vi "xy_stack_setup.vi"() -> ()   [LabVIEW 2016]
uses:
  xy_stack_global.vi
  MotorPosition.vi
panel:
  out "index 4":i32
  out "index 3":i32
  out "index 2":i32
  out "index 1":i32
  out "Array 2":bool[](array[boolean])
  in  "compareFOV":bool
  out "xLoc ROI":dbl
  out "yLoc ROI":dbl
  in  "LoadROIinfo":bool
  out "Image 2":dbl[][](graph)
  out "size(s)":i32[](array[numeric])
  in  "SaveROI":bool
  out "loading data":bool
  in  "LoadFOV":bool
  in  "String 4":string
  in  "String 3":string
  in  "String 2":string
  in  "String":string
  in  "String":string
  in  "go 5":bool
  out "save 1 y 5":dbl
  out "save 1 x 5":dbl
  in  "save 5":bool
  in  "go 4":bool
  out "save 1 y 4":dbl
  out "save 1 x 4":dbl
  in  "save 4":bool
  in  "go 3":bool
  out "save 1 y 3":dbl
  out "save 1 x 3":dbl
  in  "save 3":bool
  in  "go 2":bool
  out "save 1 y 2":dbl
  out "save 1 x 2":dbl
  in  "save 2":bool
  in  "go 1":bool
  out "save 1 y":dbl
  out "save 1 x":dbl
  in  "save 1":bool
  in  "Current MIN":bool
  out "Scan Origin":cluster{dbl, dbl}
  in  "Step Size from BS FOV":bool
  in  "Image Flipped":bool
  in  "Step Xmin":bool
  in  "Step Ymax":bool
  in  "Step Ymin":bool
  in  "Step Xmax":bool
  in  "Current MAX":bool
  in  "save":bool
  in  "update":bool
  in  "Stage to cursor":bool
  in  "New XY limits":bool
  in  "BeamScanner Scanning":bool
  out "Size new Frame":i32[](array[numeric])
  out "size array init":i32[](array[numeric])
  out "size Array IN":i32[](array[numeric])
  out "size array out":i32[](array[numeric])
  out "Frame No":u16
  in  "Latest Frame":dbl[][](array[numeric])
  out "FOV Frame":dbl(ring)=64.0 items=["4x4 µm"=0.01860032550569635, "8x8 µm"=0.0372006510113927, "16x16 µm"=0.0744013020227854, "32x32 µm"=0.1488026040455708, "64x64 µm"=0.2976052080911416, "128x128 µm"=0.5952104161822832, "256x256 µm"=1.1904208323645664, "512x512 µm"=2.380841664729133, "1024x1024 µm"=4.761683329458266, "0x0"=0.0]
  out "No. Pixels Frame":i32(ring)=128 items=["8x8"=8, "16x16"=16, "32x32"=32, "64x64"=64, "128x128"=128, "256x256"=256, "512x512"=512, "1024x1024"=1024, "optimal"=1014]
  in  "Warning Limits":dbl[][](array[numeric])=[[5000.0], [5000.0]]
  in  "Safety Limits":dbl[][](array[numeric])=[[10000.0, 100000.0], [12000.0, 62000.0]]
  in  "Write Protection":bool
  out "Image":dbl[][](graph)
  out "Travel time short":dbl
  out "Travel time long":dbl
  in  "Acceleration":dbl=10000.0 format="%#_8g"
  in  "MAX Speed":dbl=1000.0
  in  "exit":bool
  out "requested y-position":dbl=35000.0
  out "requested x-position":dbl=35000.0
  in  "Move to Y":bool
  in  "Move to X":bool
  out "# steps Y":u16=20 step=1 format="%#.0f"
  in  "Y-Maximum":dbl=35000.0 min=12000.0 max=62000.0 format="%#.2f"
  in  "Y-Minimum":dbl=33849.9 min=12000.0 max=62000.0 format="%#.2f"
  in  "Step size Y":dbl=60.0 min=0.0
  out "Y-Position":sgl format="%.2f"
  out "# steps X":u16=20 step=1 format="%#.0f"
  in  "X-Maximum":dbl=38037.9 min=10000.0 max=100000.0 format="%#.2f"
  in  "X-Minimum":dbl=38037.9 min=10000.0 max=100000.0 format="%#.2f"
  in  "Step size X":dbl=60.0 min=0.0
  out "X-Position":sgl format="%.2f"
  # "9000px * 9000 px = 4GB Ram ca, test if clever saving needed"
  # "Check velocities in KINESIS: MAYBE 10000µm/s and 100000µm/s^2"
  # "Beamscanner Settings"
  # "dX relative to start"
  # "Xmin, Xmax"
  # "SETUP"
  # "Ymin, Ymax"
  # "dY relative to start"
  # "!!! Arbitrary, assumes Objective is centrally)\n(Objective Might leave Microscope Slide/Petri Dish)"
  # "Enter values from Kinesis \nto calculate imaging delay"
  # "(Objective would touch frame)"
  # "(automatic)"
  # "µm/s^2"
  # "µm/s"
  # "x"
  # "Cursors"
  # "y"
  # "Variables"
  # "Debugging"
  # "training data: \ncalc non-spectrally-imaged frames"
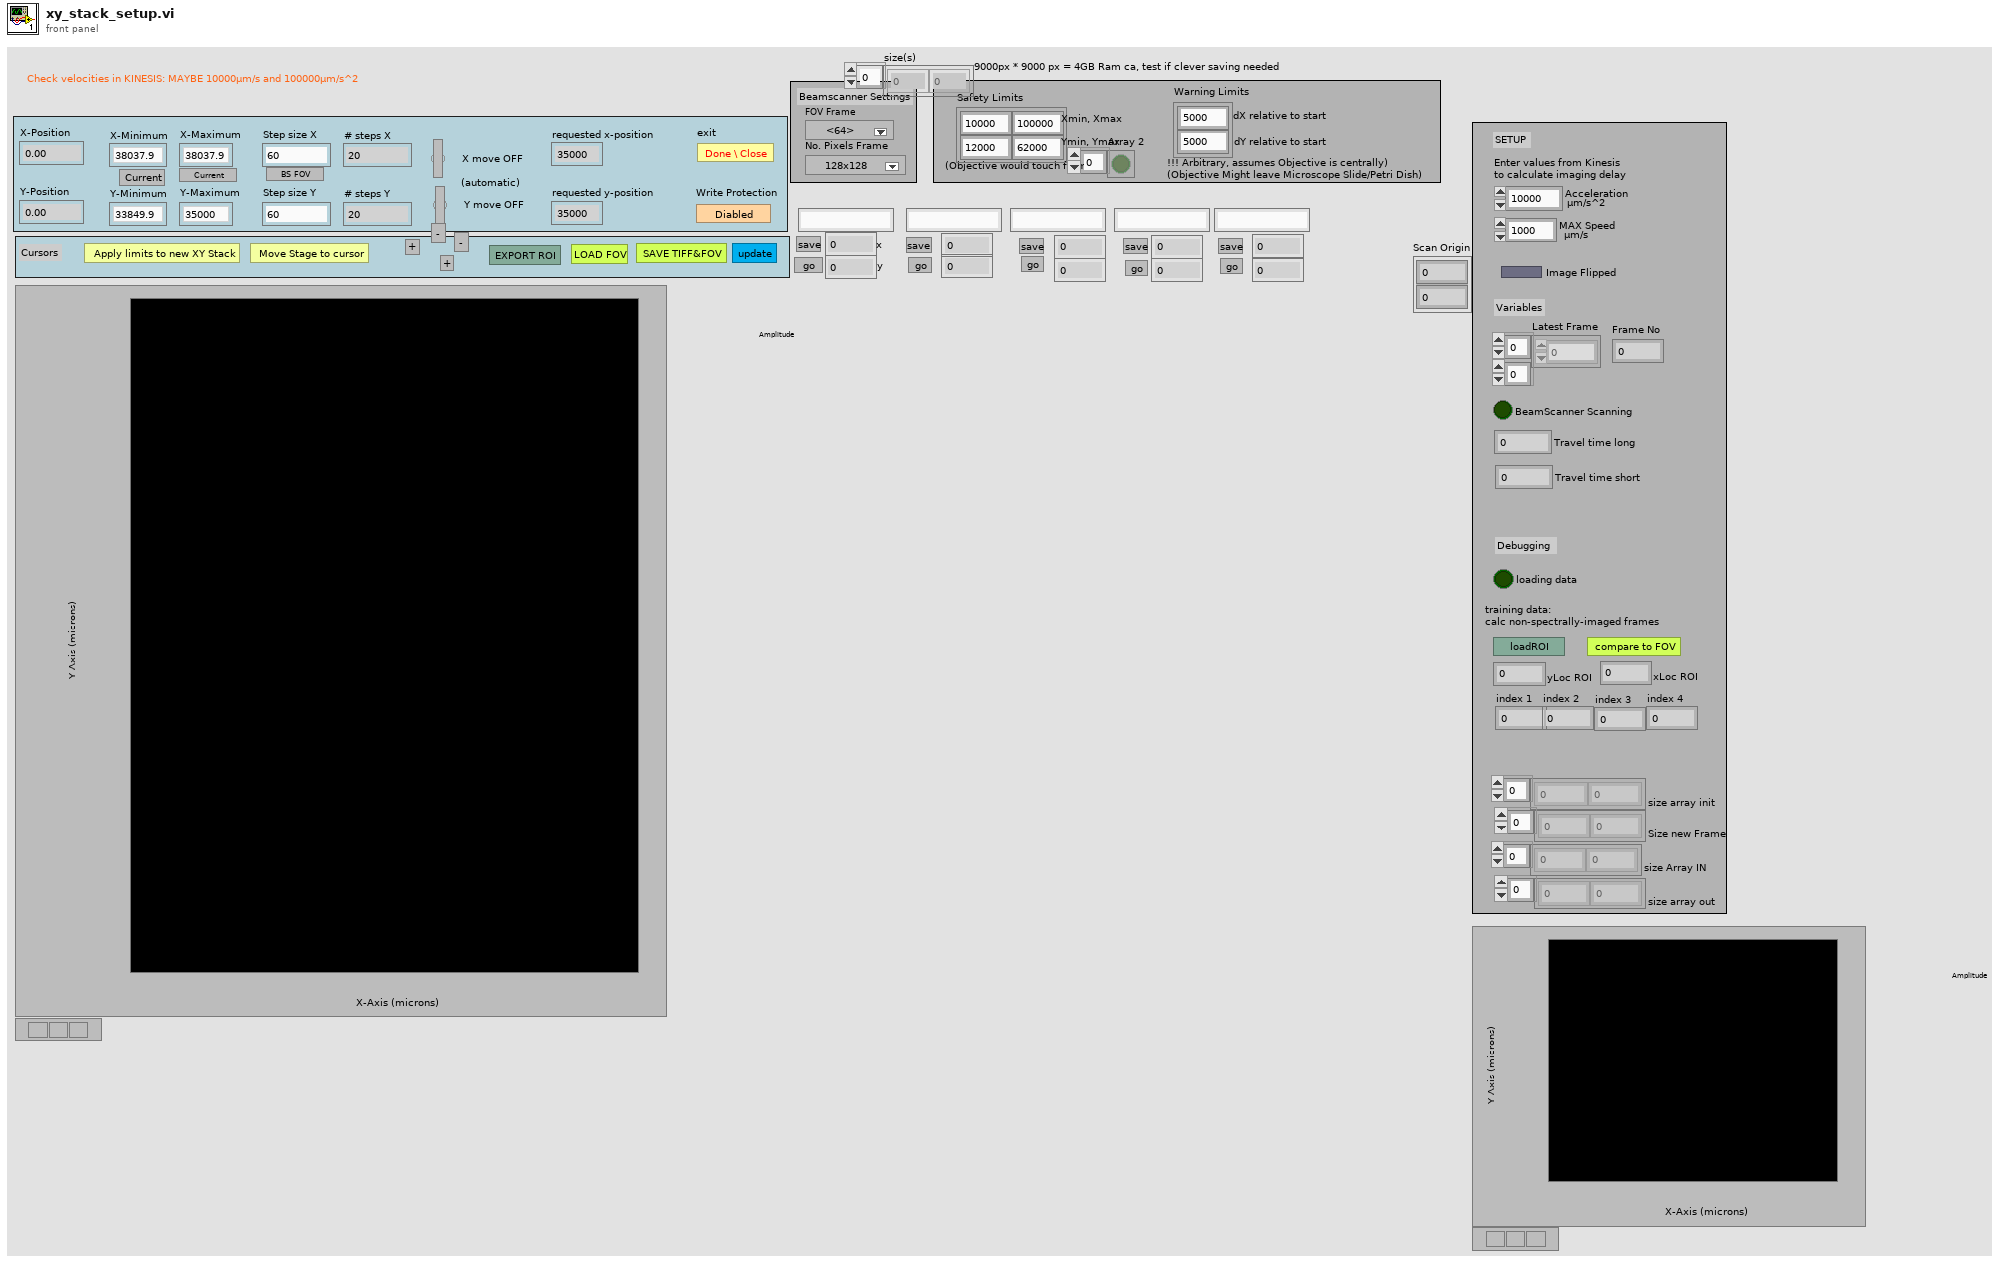
[diagram p1: front panel]
types:
  T1 = cluster{"Rows Per Strip":i32, "Photometric":i32, "Compression Type":i32}
  T2 = typedef "Image Type" = u32
  T3 = typedef "IMAQ Image.ctl" = refnum<image>
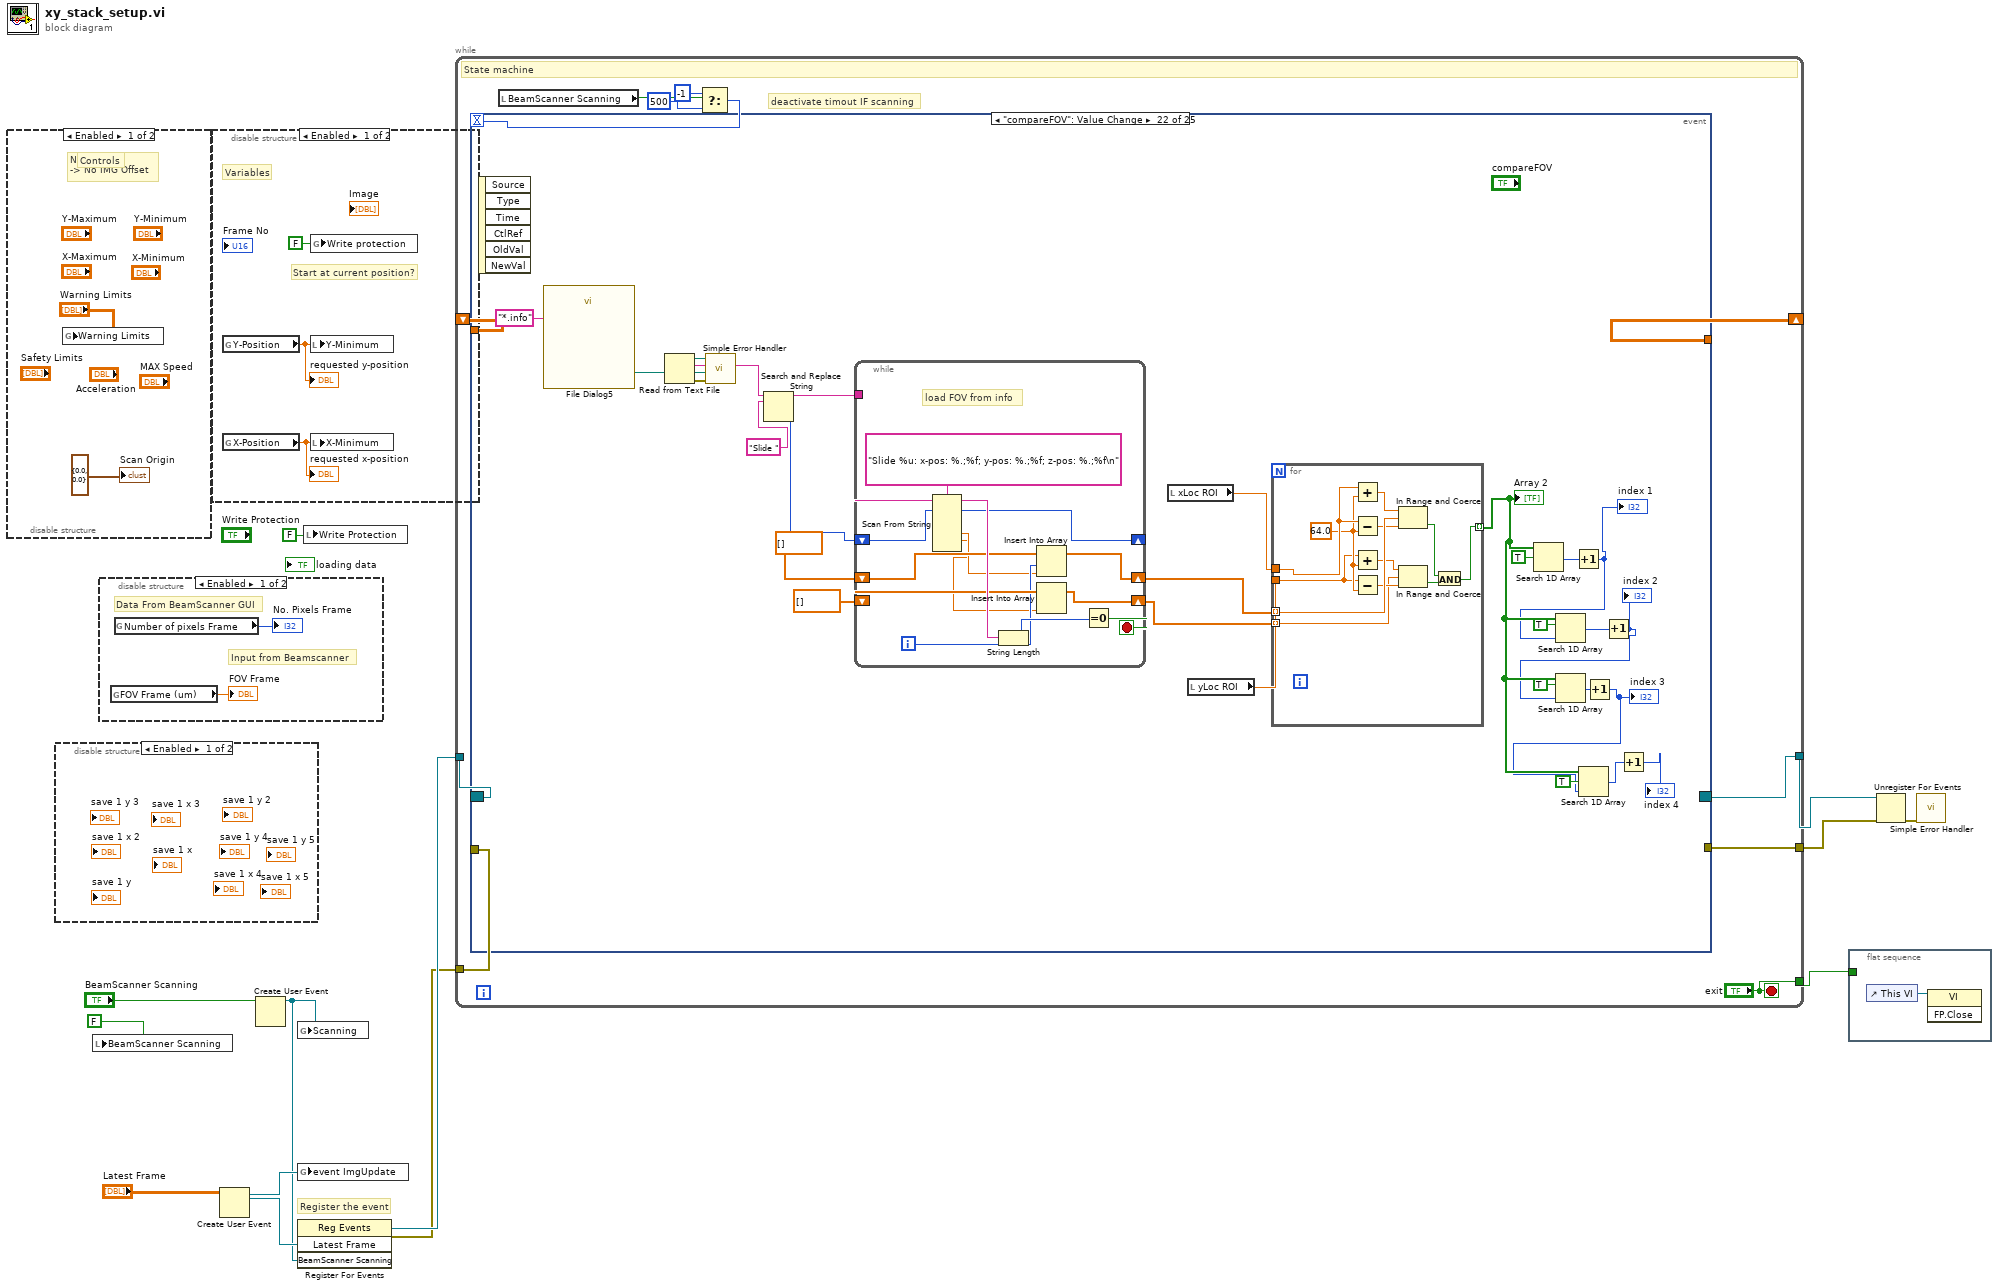
[diagram p0: block diagram]
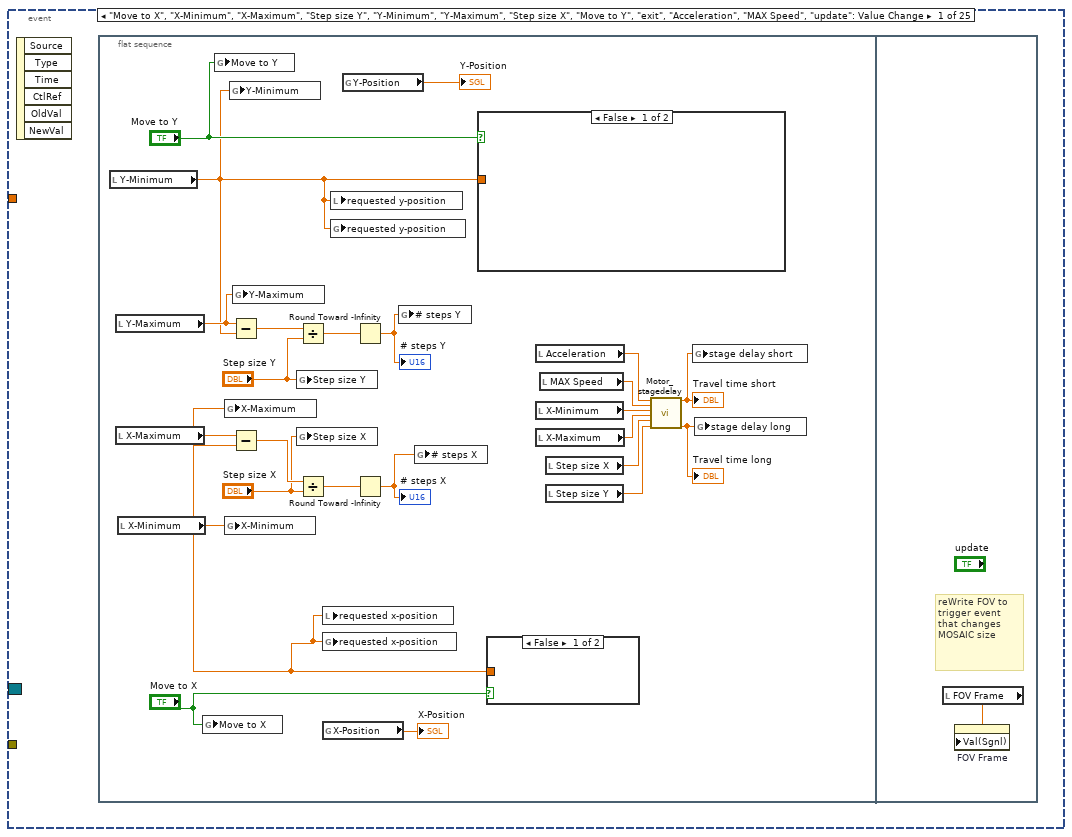
[diagram p2: hidden frame]
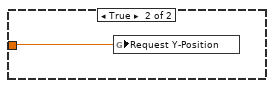
[diagram p3: hidden frame]
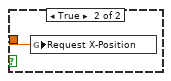
[diagram p4: hidden frame]
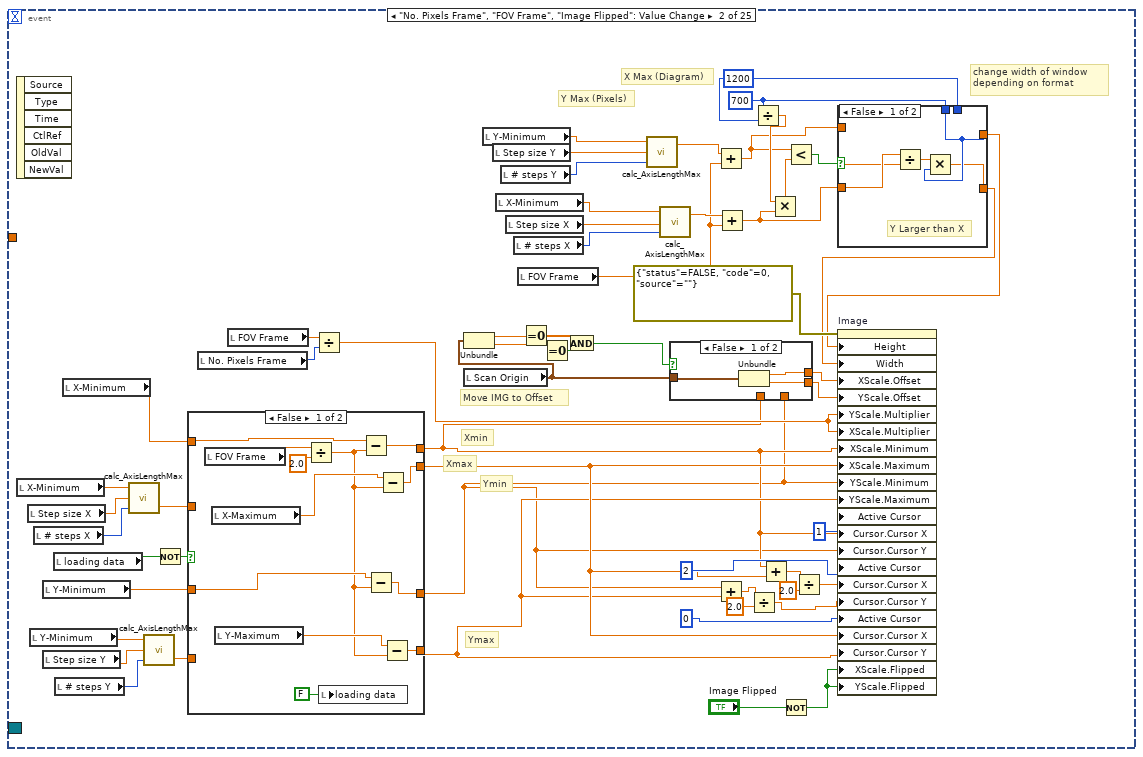
[diagram p5: hidden frame]
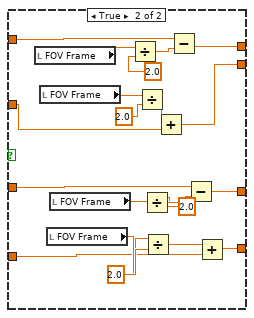
[diagram p6: hidden frame]
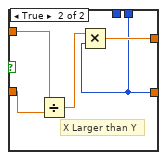
[diagram p8: hidden frame]
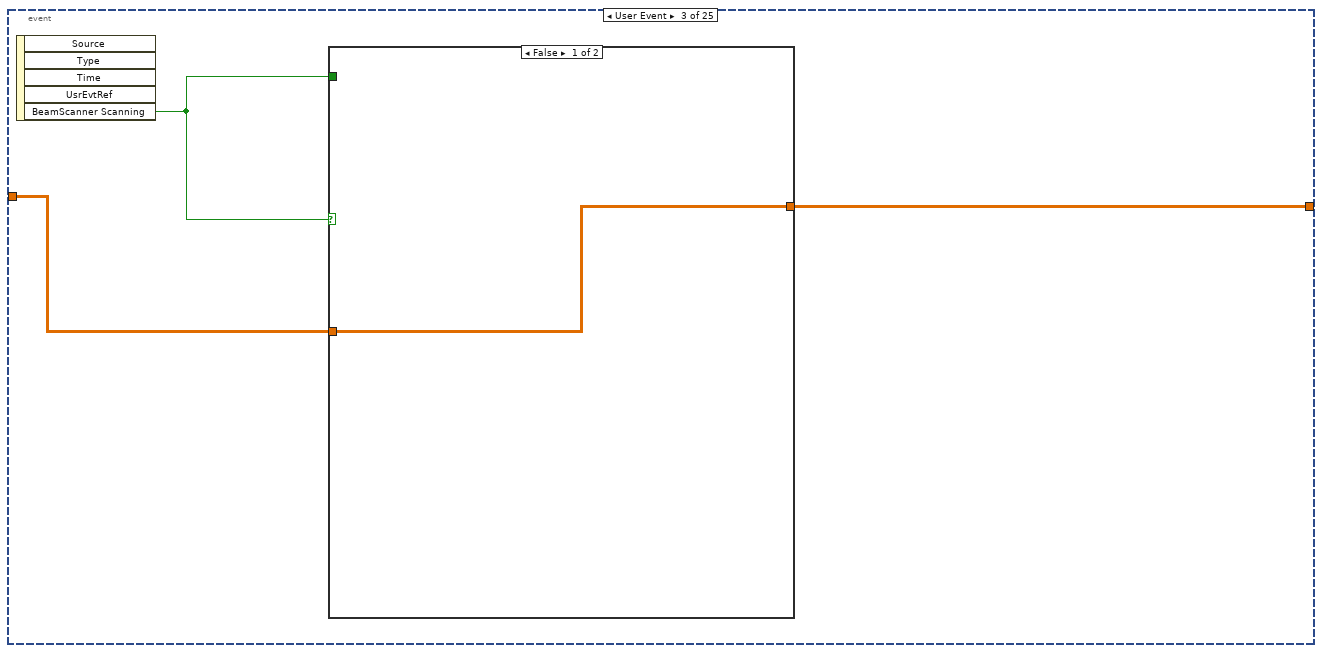
[diagram p9: hidden frame]
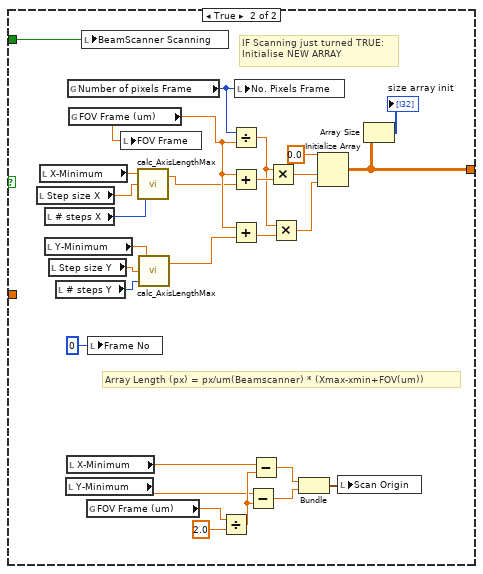
[diagram p10: hidden frame]
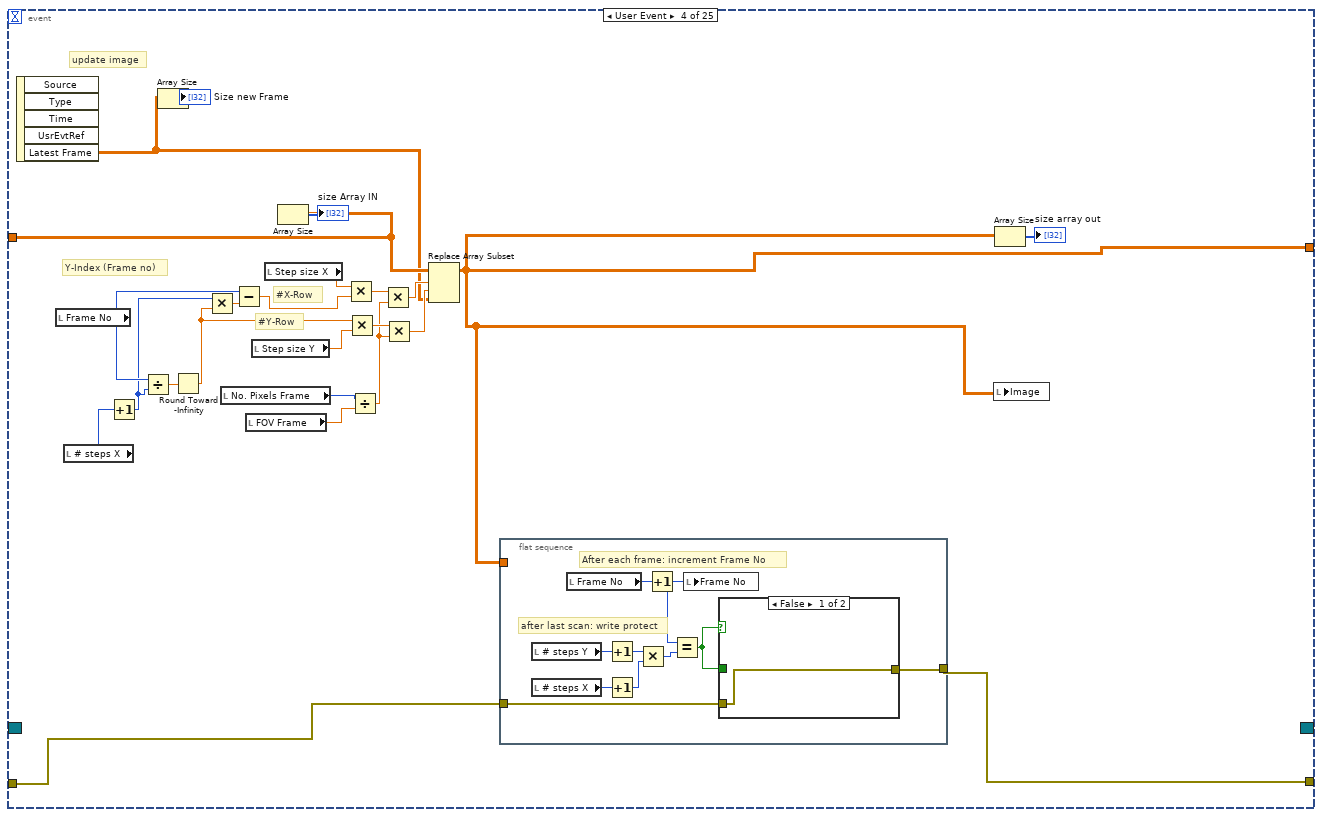
[diagram p11: hidden frame]
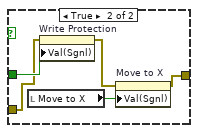
[diagram p12: hidden frame]
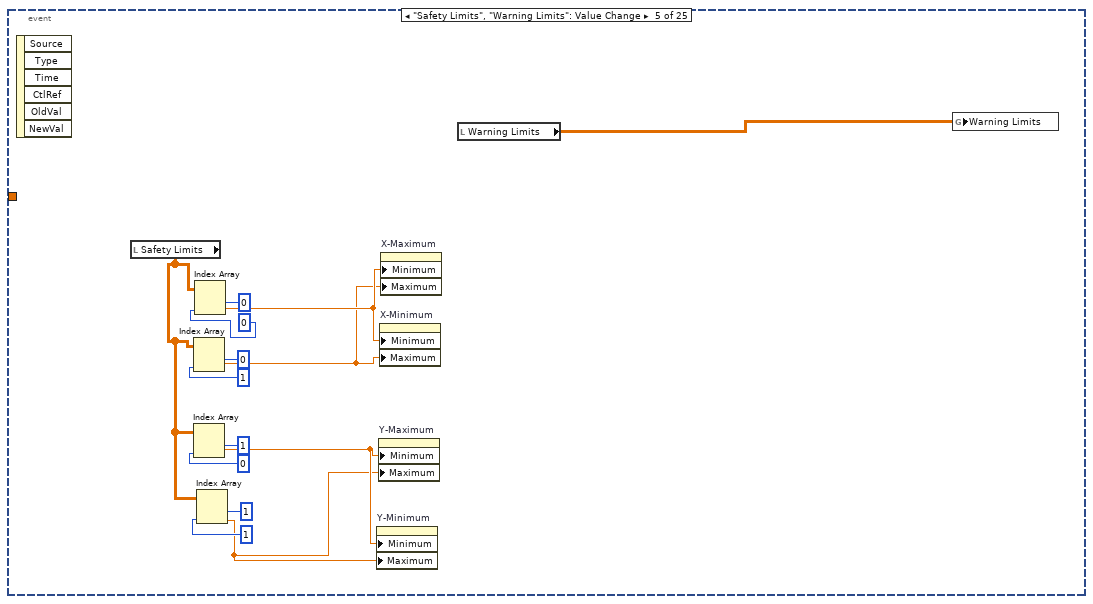
[diagram p13: hidden frame]
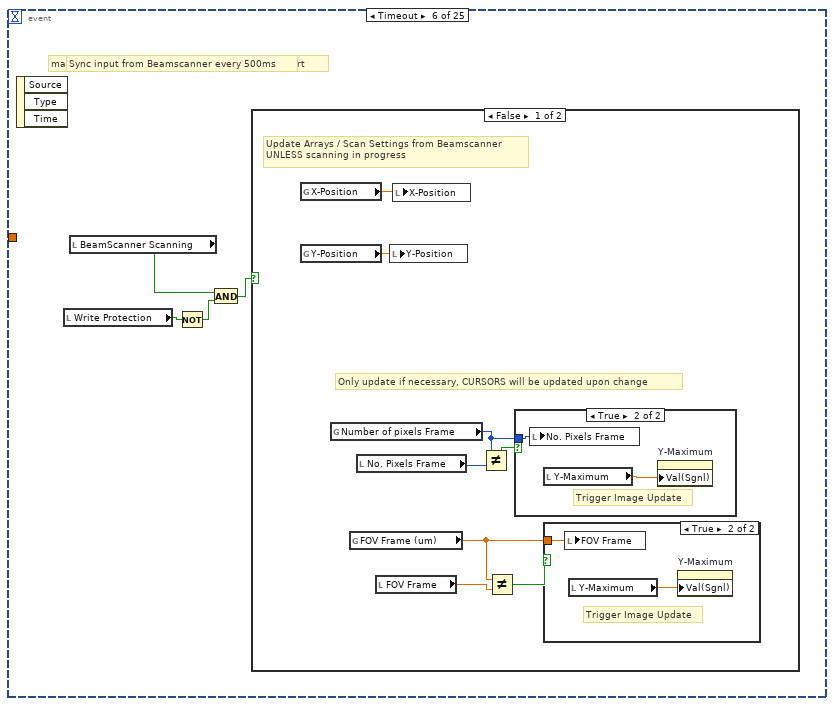
[diagram p14: hidden frame]
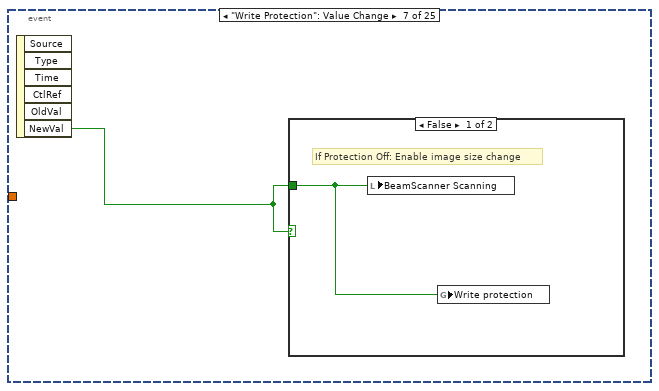
[diagram p18: hidden frame]
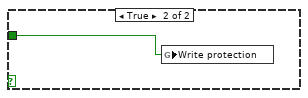
[diagram p19: hidden frame]
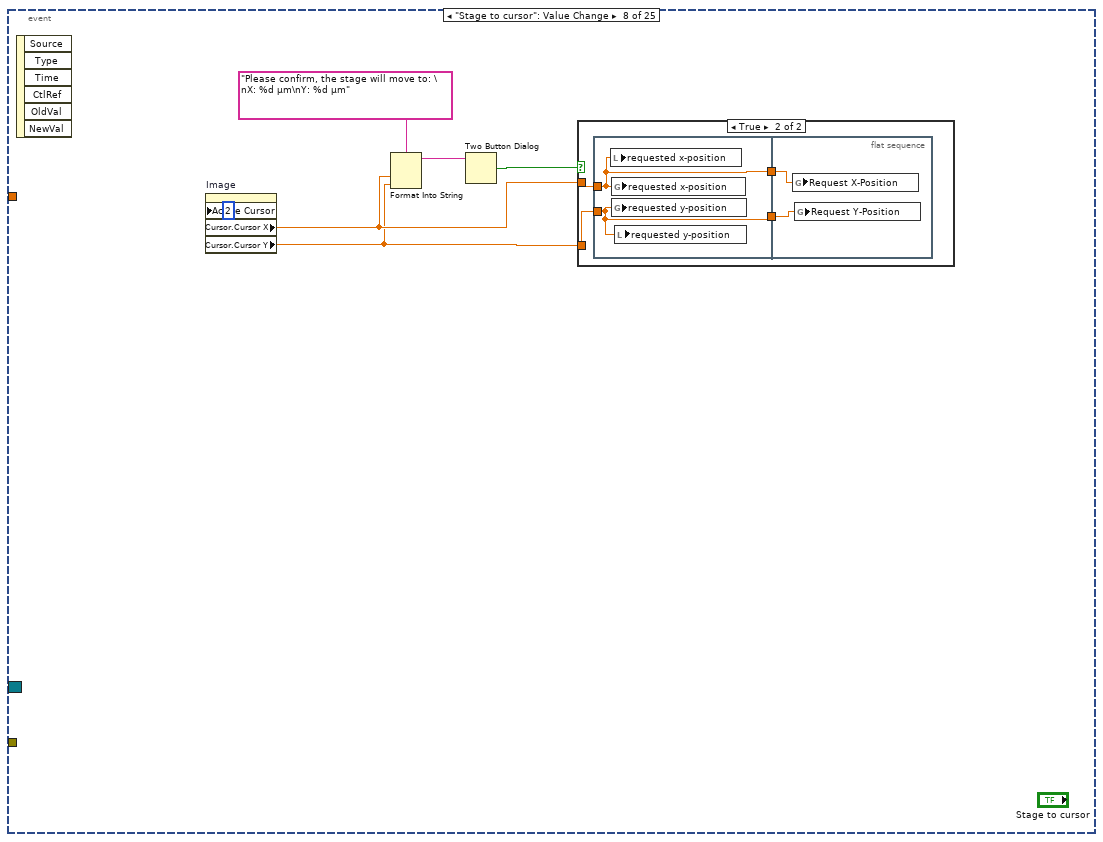
[diagram p20: hidden frame]
diagram:
  # "Register the event"
  n1 = disable-structure shown="Enabled" {
    frame Enabled {
      # "No Scan\n-> No IMG Offset"
      # "Controls"
      n2 = global write "xy_stack_global.vi" "Warning Limits"("Warning Limits") -> ()
      "Scan Origin" <- cluster{dbl, dbl} {0.0, 0.0} ("Scan Origin")
    }
    frame Disabled {
    }
  }
  n3 = disable-structure shown="Enabled" {
    frame Enabled {
    }
    frame Disabled {
    }
  }
  n4 = local write "BeamScanner Scanning"(FALSE ("BeamScanner Scanning")) -> ()
  n5 = disable-structure shown="Enabled" {
    frame Enabled {
      # "Data From BeamScanner GUI"
      # "Input from Beamscanner"
      n6 = global read "xy_stack_global.vi" "FOV Frame (um)"() -> (→"FOV Frame":dbl)
      n7 = global read "xy_stack_global.vi" "Number of pixels Frame"() -> (→"No. Pixels Frame":i32)
    }
    frame Disabled {
    }
  }
  n8 = disable-structure shown="Enabled" {
    frame Enabled {
      # "Start at current position?"
      # "Variables"
      n9 = global read "MotorPosition.vi" "Y-Position"() -> (w18:dbl)
      "requested y-position" <- w18
      n10 = global read "MotorPosition.vi" "X-Position"() -> (w19:dbl)
      "requested x-position" <- w19
      n11 = local write "Y-Minimum"(w18) -> ()
      n12 = local write "X-Minimum"(w19) -> ()
      n13 = global write "xy_stack_global.vi" "Write protection"(FALSE ("Write protection")) -> ()
    }
    frame Disabled {
    }
  }
  n14 = Create User Event(user event datatype="Latest Frame") -> (user event=w11:refnum<user-event>)  [unwired: 1 in, 1 out]
  n15 = Create User Event(user event datatype="BeamScanner Scanning") -> (user event=w3:refnum<user-event>)  [unwired: 1 in, 1 out]
  n16 = global write "xy_stack_global.vi" "Scanning"(w3) -> ()
  n17 = global write "xy_stack_global.vi" "event ImgUpdate"(w11) -> ()
  n18 = register-events(w11, w3) -> (reference out=w10:refnum<event-registration>, error out=w6:errorcluster)  [unwired: 2 in]
  n19 = local write "Write Protection"(FALSE ("New Acqusition")) -> ()
  n20 = while {
    tunnel: ["exit"] -> w12
    tunnel: w10 -> [w29]
    shift-right: [w28] -> _
    shift-left: _ -> [w27]
    tunnel: [w20] -> w7
    tunnel: w6 -> [w21]
    tunnel: [w26] -> w4
    stop <- "exit" stop-if-true
    # "deactivate timout IF scanning"
    # "State machine"
    n21 = local read "BeamScanner Scanning"() -> (w25:bool)
    n22 = Select(t=-1, s=w25, f=500) -> (s? t:f=w22:i32)
    n23 = event shown="[21] \"compareFOV\": Value Change" {
      selector: w29 -> [_ _ _ _ _ _ _ _ _ _ _ _ _ _ _ _ _ _ _ _ _ _ _ _ _]
      dyn-events: [_ _ _ _ _ _ _ _ _ _ _ _ _ _ _ _ _ _ _ _ _ _ _ _ _] -> w26
      timeout: w22 -> [_ _ _ _ _ _ _ _ _ _ _ _ _ _ _ _ _ _ _ _ _ _ _ _ _]
      tunnel: [_ _ w164 w196 _ _ _ _ _ _ _ _ _ _ _ _ _ _ _ _ w393 _ _ _ _] -> w28
      tunnel: w27 -> [_ _ w163 w209 _ _ _ _ _ _ _ _ _ _ _ _ _ _ _ _ _ _ _ _ _]
      tunnel: w21 -> [_ _ _ w194 _ _ _ _ _ _ _ _ _ _ _ _ _ _ _ _ _ _ _ _ w549]
      tunnel: [_ _ _ w195 _ _ _ _ _ _ _ _ _ _ _ _ _ _ _ _ w423 _ w521 _ w549] -> w20
      event "Move to X", "X-Minimum", "X-Maximum", "Step size Y", "Y-Minimum", "Y-Maximum", "Step size X", "Move to Y", "exit", "Acceleration", "MAX Speed", "update": Value Change {
        n24 = event-data() -> ()  [unwired: 1 in, 6 out]
        n25 = flat-sequence {
          frame #0 {
            n26 = local read "Y-Minimum"() -> (w32:dbl)
            n27 = local read "Y-Maximum"() -> (w41:dbl)
            n28 = local read "X-Maximum"() -> (w45:dbl)
            n29 = local read "X-Minimum"() -> (w31:dbl)
            n30 = global write "xy_stack_global.vi" "Move to X"("Move to X") -> ()
            n31 = global write "xy_stack_global.vi" "Move to Y"("Move to Y") -> ()
            n32 = global write "xy_stack_global.vi" "X-Maximum"(w45) -> ()
            n33 = global write "xy_stack_global.vi" "X-Minimum"(w31) -> ()
            n34 = global write "xy_stack_global.vi" "Y-Minimum"(w32) -> ()
            n35 = Subtract(x=w41, y=w32) -> (x-y=w52:dbl)
            n36 = Subtract(x=w45, y=w31) -> (x-y=w54:dbl)
            n37 = global write "xy_stack_global.vi" "Y-Maximum"(w41) -> ()
            n38 = global write "xy_stack_global.vi" "Step size Y"("Step size Y") -> ()
            n39 = global write "xy_stack_global.vi" "Step size X"("Step size X") -> ()
            n40 = Divide(x=w52, y="Step size Y") -> (x/y=w51:dbl)
            n41 = Divide(x=w54, y="Step size X") -> (x/y=w53:dbl)
            n42 = local write "requested x-position"(w31) -> ()
            n43 = global write "xy_stack_global.vi" "requested x-position"(w31) -> ()
            n44 = global read "MotorPosition.vi" "X-Position"() -> (→"X-Position":dbl)
            n45 = local write "requested y-position"(w32) -> ()
            n46 = global write "xy_stack_global.vi" "requested y-position"(w32) -> ()
            n47 = global read "MotorPosition.vi" "Y-Position"() -> (→"Y-Position":dbl)
            n48 = Round Toward -Infinity(1:w51) -> (0:w48:dbl)
            "# steps Y" <- w48
            n49 = Round Toward -Infinity(1:w53) -> (0:w50:dbl)
            "# steps X" <- w50
            n50 = global write "xy_stack_global.vi" "# steps Y"(w48) -> ()
            n51 = global write "xy_stack_global.vi" "# steps X"(w50) -> ()
            n52 = case shown="False" "Move to Y" {
              tunnel: w32 -> [_ w55]
              frame False {
              }
              frame True {
                n53 = global write "MotorPosition.vi" "Request Y-Position"(w55) -> ()
              }
            }
            n54 = case shown="False" "Move to X" {
              tunnel: w31 -> [_ w56]
              frame False {
              }
              frame True {
                n55 = global write "MotorPosition.vi" "Request X-Position"(w56) -> ()
              }
            }
            n56 = local read "Acceleration"() -> (w40:dbl)
            n57 = local read "X-Minimum"() -> (w38:dbl)
            n58 = local read "X-Maximum"() -> (w35:dbl)
            n59 = local read "MAX Speed"() -> (w39:dbl)
            n60 = local read "Step size X"() -> (w37:dbl)
            n61 = local read "Step size Y"() -> (w36:dbl)
            n62 = call "Motor_stagedelay.vi"("Acceleration"=w40, "MAX Speed"=w39, "Min X"=w38, "Max X"=w35, "Step size Y"=w37, "Step size X"=w36) -> ("Travel time short (ms)"=w34:dbl, "Travel time long (ms)"=w33:dbl)  [unwired: 12 in]
            "Travel time long" <- w33
            "Travel time short" <- w34
            n63 = global write "xy_stack_global.vi" "stage delay short"(w34) -> ()
            n64 = global write "xy_stack_global.vi" "stage delay long"(w33) -> ()
          }
          frame #1 {
            # "reWrite FOV to \ntrigger event \nthat changes \nMOSAIC size"
            n65 = local read "FOV Frame"() -> (w57:dbl)
            n66 = property on="FOV Frame" class="Ring (strict)"("Val(Sgnl)"=w57) -> ()  [unwired: 2 in, 2 out]
          }
        }
      }
      event "No. Pixels Frame", "FOV Frame", "Image Flipped": Value Change {
        w109 = u32 700 ("Plot Area:Size:Height")
        w108 = u32 1200 ("Plot Area:Size:Height")
        # "Move IMG to Offset"
        # "Xmin"
        # "Xmax"
        # "Ymin"
        # "Ymax"
        # "Y Max (Pixels)"
        # "X Max (Diagram)"
        # "change width of window \ndepending on format"
        n67 = event-data() -> ()  [unwired: 1 in, 6 out]
        n68 = local read "X-Minimum"() -> (w101:dbl)
        n69 = local read "Step size X"() -> (w100:dbl)
        n70 = local read "Y-Minimum"() -> (w97:dbl)
        n71 = local read "# steps X"() -> (w99:u16)
        n72 = local read "Y-Minimum"() -> (w113:dbl)
        n73 = local read "Step size Y"() -> (w98:dbl)
        n74 = local read "loading data"() -> (w58:bool)
        n75 = local read "# steps Y"() -> (w96:u16)
        n76 = local read "X-Minimum"() -> (w114:dbl)
        n77 = call "calc_AxisLengthMax.vi"("# steps"=w99, "Step size"=w100, "Minimum"=w101) -> ("Maximum"=w63:dbl)  [unwired: 1 out]
        n78 = call "calc_AxisLengthMax.vi"("# steps"=w96, "Step size"=w98, "Minimum"=w97) -> ("Maximum"=w62:dbl)  [unwired: 1 out]
        n79 = Not(x=w58) -> (.not. x?=w59:bool)
        n80 = case shown="False" w59 {
          tunnel: w114 -> [w124 w144]
          tunnel: w113 -> [w120 w139]
          tunnel: [w118 w134] -> w82
          tunnel: [w119 w133] -> w79
          tunnel: w63 -> [_ w132]
          tunnel: w62 -> [_ w130]
          tunnel: [w123 w128] -> w61
          tunnel: [w121 w127] -> w60
          frame False {
            n81 = local read "FOV Frame"() -> (w122:dbl)
            n82 = local read "X-Maximum"() -> (w117:dbl)
            n83 = local read "Y-Maximum"() -> (w116:dbl)
            n84 = Divide(x=w122, y=2.0) -> (x/y=w115:dbl)
            n85 = local write "loading data"(FALSE ("loading data")) -> ()
            n86 = Subtract(x=w124, y=w115) -> (x-y=w123:dbl)
            n87 = Subtract(x=w120, y=w115) -> (x-y=w121:dbl)
            n88 = Subtract(x=w117, y=w115) -> (x-y=w118:dbl)
            n89 = Subtract(x=w116, y=w115) -> (x-y=w119:dbl)
          }
          frame True {
            n90 = local read "FOV Frame"() -> (w146:dbl)
            n91 = local read "FOV Frame"() -> (w135:dbl)
            n92 = local read "FOV Frame"() -> (w137:dbl)
            n93 = local read "FOV Frame"() -> (w136:dbl)
            n94 = Divide(x=w146, y=2.0) -> (x/y=w145:dbl)
            n95 = Divide(x=w135, y=2.0) -> (x/y=w131:dbl)
            n96 = Divide(x=w136, y=2.0) -> (x/y=w141:dbl)
            n97 = Divide(x=w137, y=2.0) -> (x/y=w129:dbl)
            n98 = Add(x=w131, y=w132) -> (x+y=w134:dbl)
            n99 = Subtract(x=w144, y=w145) -> (x-y=w128:dbl)
            n100 = Subtract(x=w139, y=w141) -> (x-y=w127:dbl)
            n101 = Add(x=w129, y=w130) -> (x+y=w133:dbl)
          }
        }
        n102 = local read "No. Pixels Frame"() -> (w89:i32)
        n103 = local read "FOV Frame"() -> (w90:dbl)
        n104 = Divide(x=w90, y=w89) -> (x/y=w72:dbl)
        n105 = local read "Scan Origin"() -> (w69:cluster{dbl, dbl})
        n106 = Unbundle(w69) -> (w68:dbl, w67:dbl)
        n107 = local read "Y-Minimum"() -> (w107:dbl)
        n108 = local read "Step size Y"() -> (w106:dbl)
        n109 = local read "X-Minimum"() -> (w104:dbl)
        n110 = local read "# steps Y"() -> (w105:u16)
        n111 = local read "Step size X"() -> (w103:dbl)
        n112 = local read "# steps X"() -> (w102:u16)
        n113 = local read "FOV Frame"() -> (w93:dbl)
        n114 = Equal To 0?(x=w68) -> (x = 0?=w65:bool)
        n115 = Equal To 0?(x=w67) -> (x = 0?=w66:bool)
        n116 = And(x=w65, y=w66) -> (x .and. y?=w64:bool)
        n117 = call "calc_AxisLengthMax.vi"("# steps"=w105, "Step size"=w106, "Minimum"=w107) -> ("Length"=w94:dbl)  [unwired: 1 out]
        n118 = call "calc_AxisLengthMax.vi"("# steps"=w102, "Step size"=w103, "Minimum"=w104) -> ("Length"=w95:dbl)  [unwired: 1 out]
        n119 = case shown="False" w64 {
          tunnel: [w149 w151] -> w71
          tunnel: [w148 w150] -> w70
          tunnel: w69 -> [w147 _]
          tunnel: w61 -> [_ w151]
          tunnel: w60 -> [_ w150]
          frame False {
            n120 = Unbundle(w147) -> (w149:dbl, w148:dbl)
          }
          frame True {
            # "No Scan: Min = Offset"
          }
        }
        n121 = Add(x=w94, y=w93) -> (x+y=w92:dbl)
        n122 = Add(x=w60, y=w79) -> (x+y=w78:dbl)
        n123 = Add(x=w95, y=w93) -> (x+y=w91:dbl)
        n124 = Divide(x=w78, y=2.0) -> (x/y=w80:dbl)
        n125 = Divide(x=w109, y=w108) -> (x/y=w110:dbl)
        n126 = Add(x=w61, y=w82) -> (x+y=w85:dbl)
        n127 = Multiply(x=w110, y=w91) -> (x*y=w111:dbl)
        n128 = Not(x="Image Flipped") -> (.not. x?=w75:bool)
        n129 = Less?(x=w92, y=w111) -> (x < y?=w112:bool)
        n130 = Divide(x=w85, y=2.0) -> (x/y=w83:dbl)
        n131 = case shown="False" w112 {
          tunnel: w91 -> [w156 w161]
          tunnel: w92 -> [w155 w160]
          tunnel: [w153 w159] -> w74
          tunnel: [w152 w157] -> w73
          tunnel: w108 -> [_ w157]
          tunnel: w109 -> [w153 _]
          frame False {
            # "Y Larger than X"
            n132 = Divide(x=w156, y=w155) -> (x/y=w154:dbl)
            n133 = Multiply(x=w154, y=w153) -> (x*y=w152:dbl)
          }
          frame True {
            # "X Larger than Y"
            n134 = Divide(x=w160, y=w161) -> (x/y=w158:dbl)
            n135 = Multiply(x=w158, y=w157) -> (x*y=w159:dbl)
          }
        }
        n136 = property on="Image" class="IntGraph (strict)"(error in=errorcluster {"status"=FALSE, "code"=0, "source"=""} ("error in (no error)"), "Height"=w74, "Width"=w73, "XScale.Offset"=w71, "YScale.Offset"=w70, "YScale.Multiplier"=w72, "XScale.Multiplier"=w72, "XScale.Minimum"=w61, "XScale.Maximum"=w82, "YScale.Minimum"=w60, "YScale.Maximum"=w79, "Active Cursor"=u32 1, "Cursor.Cursor X"=w61, "Cursor.Cursor Y"=w60, "Active Cursor"=u32 2, "Cursor.Cursor X"=w83, "Cursor.Cursor Y"=w80, "Active Cursor"=u32 0, "Cursor.Cursor X"=w82, "Cursor.Cursor Y"=w79, "XScale.Flipped"=w75, "YScale.Flipped"=w75) -> ()  [unwired: 1 in, 2 out]
      }
      event User Event {
        n137 = event-data() -> ("BeamScanner Scanning"=w162:bool)  [unwired: 1 in, 4 out]
        n138 = case shown="False" w162 {
          tunnel: [w165 w193] -> w164
          tunnel: w163 -> [w165 _]
          tunnel: w162 -> [_ w189]
          frame False {
          }
          frame True {
            # "Array Length (px) = px/um(Beamscanner) * (Xmax-xmin+FOV(um))"
            # "IF Scanning just turned TRUE:\nInitialise NEW ARRAY"
            n139 = local read "Step size X"() -> (w177:dbl)
            n140 = local read "X-Minimum"() -> (w178:dbl)
            n141 = local read "# steps X"() -> (w176:u16)
            n142 = local read "Y-Minimum"() -> (w180:dbl)
            n143 = local read "Step size Y"() -> (w181:dbl)
            n144 = local read "# steps Y"() -> (w179:u16)
            n145 = local read "Y-Minimum"() -> (w169:dbl)
            n146 = local read "X-Minimum"() -> (w170:dbl)
            n147 = global read "xy_stack_global.vi" "Number of pixels Frame"() -> (w183:i32)
            n148 = global read "xy_stack_global.vi" "FOV Frame (um)"() -> (w182:dbl)
            n149 = local write "BeamScanner Scanning"(w189) -> ()
            n150 = global read "xy_stack_global.vi" "FOV Frame (um)"() -> (w172:dbl)
            n151 = local write "Frame No"(u16 0 ("Frame No")) -> ()
            n152 = local write "FOV Frame"(w182) -> ()
            n153 = call "calc_AxisLengthMax.vi"("# steps"=w176, "Step size"=w177, "Minimum"=w178) -> ("Length"=w175:dbl)  [unwired: 1 out]
            n154 = call "calc_AxisLengthMax.vi"("# steps"=w179, "Step size"=w181, "Minimum"=w180) -> ("Length"=w174:dbl)  [unwired: 1 out]
            n155 = Divide(x=w172, y=2.0) -> (x/y=w171:dbl)
            n156 = Divide(x=w183, y=w182) -> (x/y=w186:dbl)
            n157 = Add(x=w182, y=w175) -> (x+y=w188:dbl)
            n158 = Add(x=w182, y=w174) -> (x+y=w187:dbl)
            n159 = local write "No. Pixels Frame"(w183) -> ()
            n160 = Subtract(x=w169, y=w171) -> (x-y=w167:dbl)
            n161 = Subtract(x=w170, y=w171) -> (x-y=w168:dbl)
            n162 = Multiply(x=w186, y=w188) -> (x*y=w185:dbl)
            n163 = Multiply(x=w186, y=w187) -> (x*y=w184:dbl)
            n164 = Bundle(w168, w167) -> (w166:cluster{dbl, dbl})  [unwired: 1 in]
            n165 = Initialize Array(0.0, w185, w184) -> (w193:dbl[][])
            n166 = local write "Scan Origin"(w166) -> ()
            n167 = Array Size(array=w193) -> (size(s)=→"size array init":i32[])
          }
        }
      }
      event User Event {
        # "#X-Row"
        # "#Y-Row"
        # "Y-Index (Frame no)"
        # "update image"
        n168 = event-data() -> ("Latest Frame"=w197:dbl[][])  [unwired: 1 in, 4 out]
        n169 = local read "Frame No"() -> (w215:u16)
        n170 = local read "# steps X"() -> (w216:u16)
        n171 = Increment(x=w216) -> (x+1=w213:u16)
        n172 = Divide(x=w215, y=w213) -> (x/y=w217:dbl)
        n173 = Array Size(array=w197) -> (size(s)=→"Size new Frame":i32[])
        n174 = Round Toward -Infinity(1:w217) -> (0:w206:dbl)
        n175 = Multiply(x=w213, y=w206) -> (x*y=w214:dbl)
        n176 = local read "No. Pixels Frame"() -> (w199:i32)
        n177 = Subtract(x=w215, y=w214) -> (x-y=w207:dbl)
        n178 = local read "FOV Frame"() -> (w198:dbl)
        n179 = local read "Step size Y"() -> (w205:dbl)
        n180 = local read "Step size X"() -> (w208:dbl)
        n181 = Array Size(array=w209) -> (size(s)=→"size Array IN":i32[])
        n182 = Multiply(x=w208, y=w207) -> (x*y=w204:dbl)
        n183 = Multiply(x=w206, y=w205) -> (x*y=w203:dbl)
        n184 = Divide(x=w199, y=w198) -> (x/y=w202:dbl)
        n185 = Multiply(x=w204, y=w202) -> (x*y=w201:dbl)
        n186 = Multiply(x=w203, y=w202) -> (x*y=w200:dbl)
        n187 = Replace Array Subset(array=w209, new element=w197, index (row)=w201, index (col)=w200) -> (w196:dbl[][])
        n188 = flat-sequence {
          tunnel: w196 -> [_]
          tunnel: [w219] -> w195
          tunnel: w194 -> [w218]
          frame #0 {
            # "after last scan: write protect"
            # "After each frame: increment Frame No"
            n189 = local read "# steps Y"() -> (w226:u16)
            n190 = local read "# steps X"() -> (w222:u16)
            n191 = local read "Frame No"() -> (w227:u16)
            n192 = Increment(x=w226) -> (x+1=w221:u16)
            n193 = Increment(x=w222) -> (x+1=w220:u16)
            n194 = Multiply(x=w221, y=w220) -> (x*y=w224:u16)
            n195 = Increment(x=w227) -> (x+1=w225:u16)
            n196 = Equal?(x=w225, y=w224) -> (x = y?=w223:bool)
            n197 = local write "Frame No"(w225) -> ()
            n198 = case shown="False" w223 {
              tunnel: w223 -> [_ w233]
              tunnel: [w228 w230] -> w219
              tunnel: w218 -> [w228 w229]
              frame False {
              }
              frame True {
                n199 = local read "Move to X"() -> (w232:bool)
                n200 = property on="Write Protection" class="Bool (strict)"(error in=w229, "Val(Sgnl)"=w233) -> (error out=w231:errorcluster)  [unwired: 1 in, 1 out]
                n201 = property on="Move to X" class="Bool (strict)"(error in=w231, "Val(Sgnl)"=w232) -> (error out=w230:errorcluster)  [unwired: 1 in, 1 out]
              }
            }
          }
        }
        n202 = local write "Image"(w196) -> ()
        n203 = Array Size(array=w196) -> (size(s)=→"size array out":i32[])
      }
      event "Safety Limits", "Warning Limits": Value Change {
        n204 = event-data() -> ()  [unwired: 1 in, 6 out]
        n205 = local read "Safety Limits"() -> (w247:dbl[][])
        n206 = Index Array(array=w247, index (row)=0, index (col)=1 ("disabled index (col)")) -> (element=w237:dbl)
        n207 = Index Array(array=w247, index (row)=1, index (col)=0 ("disabled index (col)")) -> (element=w236:dbl)
        n208 = Index Array(array=w247, index (row)=0, index (col)=0 ("disabled index (col)")) -> (element=w238:dbl)
        n209 = Index Array(array=w247, index (row)=1, index (col)=1 ("disabled index (col)")) -> (element=w235:dbl)
        n210 = property on="Y-Minimum" class="DigNum (strict)"("Minimum"=w236, "Maximum"=w235) -> ()  [unwired: 2 in, 2 out]
        n211 = property on="Y-Maximum" class="DigNum (strict)"("Minimum"=w236, "Maximum"=w235) -> ()  [unwired: 2 in, 2 out]
        n212 = property on="X-Minimum" class="DigNum (strict)"("Minimum"=w238, "Maximum"=w237) -> ()  [unwired: 2 in, 2 out]
        n213 = property on="X-Maximum" class="DigNum (strict)"("Minimum"=w238, "Maximum"=w237) -> ()  [unwired: 2 in, 2 out]
        n214 = local read "Warning Limits"() -> (w234:dbl[][])
        n215 = global write "xy_stack_global.vi" "Warning Limits"(w234) -> ()
      }
      event Timeout {
        # "make sure event triggert by FOV and PXL are triggert"
        # "Sync input from Beamscanner every 500ms"
        n216 = event-data() -> ()  [unwired: 1 in, 3 out]
        n217 = local read "Write Protection"() -> (w249:bool)
        n218 = local read "BeamScanner Scanning"() -> (w248:bool)
        n219 = Not(x=w249) -> (.not. x?=w250:bool)
        n220 = And(x=w248, y=w250) -> (x .and. y?=w251:bool)
        n221 = case shown="False" w251 {
          frame False {
            # "Only update if necessary, CURSORS will be updated upon change"
            # "Update Arrays / Scan Settings from Beamscanner \nUNLESS scanning in progress"
            n222 = global read "MotorPosition.vi" "X-Position"() -> (w258:dbl)
            n223 = global read "MotorPosition.vi" "Y-Position"() -> (w259:dbl)
            n224 = global read "xy_stack_global.vi" "Number of pixels Frame"() -> (w257:i32)
            n225 = global read "xy_stack_global.vi" "FOV Frame (um)"() -> (w253:dbl)
            n226 = local read "No. Pixels Frame"() -> (w256:i32)
            n227 = local read "FOV Frame"() -> (w254:dbl)
            n228 = local write "Y-Position"(w259) -> ()
            n229 = local write "X-Position"(w258) -> ()
            n230 = Not Equal?(x=w257, y=w256) -> (x != y?=w255:bool)
            n231 = Not Equal?(x=w253, y=w254) -> (x != y?=w252:bool)
            n232 = case shown="True" w255 {
              tunnel: w257 -> [_ w263]
              frame False {
              }
              frame True {
                # "Trigger Image Update"
                n233 = local write "No. Pixels Frame"(w263) -> ()
                n234 = local read "Y-Maximum"() -> (w262:dbl)
                n235 = property on="Y-Maximum" class="DigNum (strict)"("Val(Sgnl)"=w262) -> ()  [unwired: 2 in, 2 out]
              }
            }
            n236 = case shown="True" w252 {
              tunnel: w253 -> [_ w261]
              frame False {
              }
              frame True {
                # "Trigger Image Update"
                n237 = local write "FOV Frame"(w261) -> ()
                n238 = local read "Y-Maximum"() -> (w260:dbl)
                n239 = property on="Y-Maximum" class="DigNum (strict)"("Val(Sgnl)"=w260) -> ()  [unwired: 2 in, 2 out]
              }
            }
          }
          frame True {
          }
        }
      }
      event "Write Protection": Value Change {
        n240 = event-data() -> ("NewVal"=w264:bool)  [unwired: 1 in, 5 out]
        n241 = case shown="False" w264 {
          tunnel: w264 -> [w265 w266]
          frame False {
            # "If Protection Off: Enable image size change"
            n242 = local write "BeamScanner Scanning"(w265) -> ()
            n243 = global write "xy_stack_global.vi" "Write protection"(w265) -> ()
          }
          frame True {
            n244 = global write "xy_stack_global.vi" "Write protection"(w266) -> ()
          }
        }
      }
      event "Stage to cursor": Value Change {
        n245 = event-data() -> ()  [unwired: 1 in, 6 out]
        n246 = property on="Image" class="IntGraph (strict)"("Active Cursor"=u32 2) -> ("Cursor.Cursor X"=w268:dbl, "Cursor.Cursor Y"=w267:dbl)  [unwired: 2 in, 2 out]
        n247 = Format Into String(format string="Please confirm, the stage will move to: \nX: %d µm\nY: %d µm" ("message"), w268, w267) -> (resulting string=w270:string)  [unwired: 2 in, 1 out]
        n248 = Two Button Dialog(message=w270) -> (T button?=w271:bool)  [unwired: 2 in]
        n249 = case shown="True" w271 {
          tunnel: w268 -> [_ w275]
          tunnel: w267 -> [_ w276]
          frame False {
          }
          frame True {
            n250 = flat-sequence {
              tunnel: w276 -> [w277]
              tunnel: w275 -> [w278]
              tunnel: [w278] -> w274
              tunnel: [w277] -> w273
              tunnel: w274 -> [w280]
              tunnel: w273 -> [w279]
              frame #0 {
                n251 = local write "requested x-position"(w278) -> ()
                n252 = global write "xy_stack_global.vi" "requested x-position"(w278) -> ()
                n253 = global write "xy_stack_global.vi" "requested y-position"(w277) -> ()
                n254 = local write "requested y-position"(w277) -> ()
              }
              frame #1 {
                n255 = global write "MotorPosition.vi" "Request X-Position"(w280) -> ()
                n256 = global write "MotorPosition.vi" "Request Y-Position"(w279) -> ()
              }
            }
          }
        }
      }
      event "go 1": Value Change {
        n257 = event-data() -> ()  [unwired: 1 in, 6 out]
        n258 = local read "save 1 x"() -> (w282:dbl)
        n259 = local read "save 1 y"() -> (w281:dbl)
        n260 = Format Into String(format string="Please confirm, the stage will move to: \nX: %d µm\nY: %d µm" ("message"), w282, w281) -> (resulting string=w284:string)  [unwired: 2 in, 1 out]
        n261 = Two Button Dialog(message=w284) -> (T button?=w285:bool)  [unwired: 2 in]
        n262 = case shown="True" w285 {
          tunnel: w282 -> [_ w288]
          tunnel: w281 -> [_ w289]
          frame False {
          }
          frame True {
            n263 = flat-sequence {
              tunnel: w289 -> [w290]
              tunnel: w288 -> [w291]
              tunnel: [w291] -> w287
              tunnel: [w290] -> w286
              tunnel: w287 -> [w293]
              tunnel: w286 -> [w292]
              frame #0 {
                n264 = local write "requested x-position"(w291) -> ()
                n265 = global write "xy_stack_global.vi" "requested x-position"(w291) -> ()
                n266 = global write "xy_stack_global.vi" "requested y-position"(w290) -> ()
                n267 = local write "requested y-position"(w290) -> ()
              }
              frame #1 {
                n268 = global write "MotorPosition.vi" "Request X-Position"(w293) -> ()
                n269 = global write "MotorPosition.vi" "Request Y-Position"(w292) -> ()
              }
            }
          }
        }
      }
      event "save 1": Value Change {
        n270 = event-data() -> ()  [unwired: 1 in, 6 out]
        n271 = global read "MotorPosition.vi" "Y-Position"() -> (w294:dbl)
        n272 = global read "MotorPosition.vi" "X-Position"() -> (w295:dbl)
        n273 = local write "save 1 x"(w295) -> ()
        n274 = local write "save 1 y"(w294) -> ()
      }
      event "save 2": Value Change {
        n275 = event-data() -> ()  [unwired: 1 in, 6 out]
        n276 = global read "MotorPosition.vi" "Y-Position"() -> (w296:dbl)
        n277 = global read "MotorPosition.vi" "X-Position"() -> (w297:dbl)
        n278 = local write "save 1 y 2"(w296) -> ()
        n279 = local write "save 1 x 2"(w297) -> ()
      }
      event "save 3": Value Change {
        n280 = event-data() -> ()  [unwired: 1 in, 6 out]
        n281 = global read "MotorPosition.vi" "Y-Position"() -> (w298:dbl)
        n282 = global read "MotorPosition.vi" "X-Position"() -> (w299:dbl)
        n283 = local write "save 1 y 3"(w298) -> ()
        n284 = local write "save 1 x 3"(w299) -> ()
      }
      event "save 4": Value Change {
        n285 = event-data() -> ()  [unwired: 1 in, 6 out]
        n286 = global read "MotorPosition.vi" "Y-Position"() -> (w300:dbl)
        n287 = global read "MotorPosition.vi" "X-Position"() -> (w301:dbl)
        n288 = local write "save 1 y 4"(w300) -> ()
        n289 = local write "save 1 x 4"(w301) -> ()
      }
      event "save 5": Value Change {
        n290 = event-data() -> ()  [unwired: 1 in, 6 out]
        n291 = global read "MotorPosition.vi" "Y-Position"() -> (w302:dbl)
        n292 = global read "MotorPosition.vi" "X-Position"() -> (w303:dbl)
        n293 = local write "save 1 y 5"(w302) -> ()
        n294 = local write "save 1 x 5"(w303) -> ()
      }
      event "go 2": Value Change {
        n295 = event-data() -> ()  [unwired: 1 in, 6 out]
        n296 = local read "save 1 y 2"() -> (w304:dbl)
        n297 = local read "save 1 x 2"() -> (w305:dbl)
        n298 = Format Into String(format string="Please confirm, the stage will move to: \nX: %d µm\nY: %d µm" ("message"), w305, w304) -> (resulting string=w307:string)  [unwired: 2 in, 1 out]
        n299 = Two Button Dialog(message=w307) -> (T button?=w308:bool)  [unwired: 2 in]
        n300 = case shown="True" w308 {
          tunnel: w305 -> [_ w311]
          tunnel: w304 -> [_ w312]
          frame False {
          }
          frame True {
            n301 = flat-sequence {
              tunnel: w312 -> [w313]
              tunnel: w311 -> [w314]
              tunnel: [w314] -> w310
              tunnel: [w313] -> w309
              tunnel: w310 -> [w316]
              tunnel: w309 -> [w315]
              frame #0 {
                n302 = local write "requested x-position"(w314) -> ()
                n303 = global write "xy_stack_global.vi" "requested x-position"(w314) -> ()
                n304 = global write "xy_stack_global.vi" "requested y-position"(w313) -> ()
                n305 = local write "requested y-position"(w313) -> ()
              }
              frame #1 {
                n306 = global write "MotorPosition.vi" "Request X-Position"(w316) -> ()
                n307 = global write "MotorPosition.vi" "Request Y-Position"(w315) -> ()
              }
            }
          }
        }
      }
      event "go 3": Value Change {
        n308 = event-data() -> ()  [unwired: 1 in, 6 out]
        n309 = local read "save 1 y 3"() -> (w317:dbl)
        n310 = local read "save 1 x 3"() -> (w318:dbl)
        n311 = Format Into String(format string="Please confirm, the stage will move to: \nX: %d µm\nY: %d µm" ("message"), w318, w317) -> (resulting string=w320:string)  [unwired: 2 in, 1 out]
        n312 = Two Button Dialog(message=w320) -> (T button?=w321:bool)  [unwired: 2 in]
        n313 = case shown="True" w321 {
          tunnel: w318 -> [_ w324]
          tunnel: w317 -> [_ w325]
          frame False {
          }
          frame True {
            n314 = flat-sequence {
              tunnel: w325 -> [w326]
              tunnel: w324 -> [w327]
              tunnel: [w327] -> w323
              tunnel: [w326] -> w322
              tunnel: w323 -> [w329]
              tunnel: w322 -> [w328]
              frame #0 {
                n315 = local write "requested x-position"(w327) -> ()
                n316 = global write "xy_stack_global.vi" "requested x-position"(w327) -> ()
                n317 = global write "xy_stack_global.vi" "requested y-position"(w326) -> ()
                n318 = local write "requested y-position"(w326) -> ()
              }
              frame #1 {
                n319 = global write "MotorPosition.vi" "Request X-Position"(w329) -> ()
                n320 = global write "MotorPosition.vi" "Request Y-Position"(w328) -> ()
              }
            }
          }
        }
      }
      event "go 4": Value Change {
        n321 = event-data() -> ()  [unwired: 1 in, 6 out]
        n322 = local read "save 1 y 4"() -> (w330:dbl)
        n323 = local read "save 1 x 4"() -> (w331:dbl)
        n324 = Format Into String(format string="Please confirm, the stage will move to: \nX: %d µm\nY: %d µm" ("message"), w331, w330) -> (resulting string=w333:string)  [unwired: 2 in, 1 out]
        n325 = Two Button Dialog(message=w333) -> (T button?=w334:bool)  [unwired: 2 in]
        n326 = case shown="True" w334 {
          tunnel: w331 -> [_ w337]
          tunnel: w330 -> [_ w338]
          frame False {
          }
          frame True {
            n327 = flat-sequence {
              tunnel: w338 -> [w339]
              tunnel: w337 -> [w340]
              tunnel: [w340] -> w336
              tunnel: [w339] -> w335
              tunnel: w336 -> [w342]
              tunnel: w335 -> [w341]
              frame #0 {
                n328 = local write "requested x-position"(w340) -> ()
                n329 = global write "xy_stack_global.vi" "requested x-position"(w340) -> ()
                n330 = global write "xy_stack_global.vi" "requested y-position"(w339) -> ()
                n331 = local write "requested y-position"(w339) -> ()
              }
              frame #1 {
                n332 = global write "MotorPosition.vi" "Request X-Position"(w342) -> ()
                n333 = global write "MotorPosition.vi" "Request Y-Position"(w341) -> ()
              }
            }
          }
        }
      }
      event "go 5": Value Change {
        n334 = event-data() -> ()  [unwired: 1 in, 6 out]
        n335 = local read "save 1 y 5"() -> (w343:dbl)
        n336 = local read "save 1 x 5"() -> (w344:dbl)
        n337 = Format Into String(format string="Please confirm, the stage will move to: \nX: %d µm\nY: %d µm" ("message"), w344, w343) -> (resulting string=w346:string)  [unwired: 2 in, 1 out]
        n338 = Two Button Dialog(message=w346) -> (T button?=w347:bool)  [unwired: 2 in]
        n339 = case shown="True" w347 {
          tunnel: w344 -> [_ w350]
          tunnel: w343 -> [_ w351]
          frame False {
          }
          frame True {
            n340 = flat-sequence {
              tunnel: w351 -> [w352]
              tunnel: w350 -> [w353]
              tunnel: [w353] -> w349
              tunnel: [w352] -> w348
              tunnel: w349 -> [w355]
              tunnel: w348 -> [w354]
              frame #0 {
                n341 = local write "requested x-position"(w353) -> ()
                n342 = global write "xy_stack_global.vi" "requested x-position"(w353) -> ()
                n343 = global write "xy_stack_global.vi" "requested y-position"(w352) -> ()
                n344 = local write "requested y-position"(w352) -> ()
              }
              frame #1 {
                n345 = global write "MotorPosition.vi" "Request X-Position"(w355) -> ()
                n346 = global write "MotorPosition.vi" "Request Y-Position"(w354) -> ()
              }
            }
          }
        }
      }
      event "New XY limits": Value Change {
        n347 = event-data() -> ()  [unwired: 1 in, 6 out]
        n348 = property on="Image" class="IntGraph (strict)"("Active Cursor"=u32 1, "Active Cursor"=u32 0) -> ("Cursor.Cursor X"=w364:dbl, "Cursor.Cursor Y"=w363:dbl, "Cursor.Cursor X"=w362:dbl, "Cursor.Cursor Y"=w361:dbl)  [unwired: 2 in, 2 out]
        n349 = Format Into String(format string="Please confirm new limits: \nXmin: %d µm\nYmin: %d µm\nXmax: %d µm\nYmax: %d µm\nBuffer will be released for new acquisition." ("message"), w364, w363, w362, w361) -> (resulting string=w367:string)  [unwired: 2 in, 1 out]
        n350 = local read "FOV Frame"() -> (w358:dbl)
        n351 = Two Button Dialog(message=w367) -> (T button?=w360:bool)  [unwired: 2 in]
        n352 = Divide(x=w358, y=2.0) -> (x/y=w357:dbl)
        n353 = case shown="True" w360 {
          tunnel: w364 -> [_ w376]
          tunnel: w363 -> [_ w375]
          tunnel: w362 -> [_ w374]
          tunnel: w361 -> [_ w373]
          tunnel: w357 -> [_ w377]
          frame False {
          }
          frame True {
            n354 = Add(x=w376, y=w377) -> (x+y=w370:dbl)
            n355 = Subtract(x=w374, y=w377) -> (x-y=w372:dbl)
            n356 = Subtract(x=w373, y=w377) -> (x-y=w369:dbl)
            n357 = Add(x=w375, y=w377) -> (x+y=w371:dbl)
            n358 = local write "X-Minimum"(w370) -> ()
            n359 = local write "Y-Minimum"(w371) -> ()
            n360 = local write "X-Maximum"(w372) -> ()
            n361 = local write "Y-Maximum"(w369) -> ()
            n362 = property on="Y-Maximum" class="DigNum (strict)"("Val(Sgnl)"=w369) -> ()  [unwired: 2 in, 2 out]
          }
        }
        n363 = property on="Write Protection" class="Bool (strict)"("Val(Sgnl)"=FALSE ("Value (Signaling)")) -> ()  [unwired: 2 in, 2 out]
      }
      event "save": Value Change {
        # "empty array disables retrace"
        n364 = event-data() -> ()  [unwired: 1 in, 6 out]
        n365 = call "File Dialog"() -> ("selected path"=w380:path)  [unwired: 12 in, 3 out]
        n366 = Path To String(path=w380) -> (string=w381:string)
        n367 = global read "xy_stack_global.vi" "Info file content"() -> (w385:string)
        n368 = local read "Image"() -> (w378:dbl[][])
        n369 = Concatenate Strings(w381, "_MOSAIC_" ("string")) -> (w384:string)
        n370 = String To Path(string=w384) -> (path=w382:path)
        n371 = call "save_to_disk.vi"("Retrace"=dbl[][] [], "write info file?"=TRUE, "Scan info"=w385, "Image"=w378, "File path"=w382) -> ()  [unwired: 4 in, 1 out]
      }
      event "LoadFOV": Value Change {
        w420 = T2 1 items=["Grayscale (U8)", "Grayscale (I16)", "Grayscale (SGL)", "Complex (CSG)", "RGB (U32)", "HSL (U32)", "RGB (U64)", "Grayscale (U16)"] ("Image Type")
        # "img size X"
        # "img size Y"
        # "um/pixel"
        # "load FOV from info"
        n372 = event-data() -> ()  [unwired: 1 in, 6 out]
        n373 = call "File Dialog2"("pattern (all files)"="*.tiff") -> ("selected path"=w396:path, "error out"=w425:errorcluster)  [unwired: 11 in, 2 out]
        n374 = Path To String(path=w396) -> (string=w419:string)
        n375 = Search and Replace String(input string=w419, search string="_0.tiff", replace string=".info" ("replace string (\"\")")) -> (result string=w416:string, number of replacements=w390:i32, error out=w415:errorcluster)  [unwired: 5 in, 1 out]
        n376 = String To Path(string=w416) -> (path=w414:path)
        n377 = call <vilib>:"Simple Error Handler.vi"("error in (no error)"=w415) -> ()  [unwired: 4 in, 5 out]
        n378 = Greater Than 0?(x=w390) -> (x > 0?=w387:bool)
        n379 = call <vilib>:"Check if File or Folder Exists.vi"("path"=w414) -> ("file or folder exists?"=w388:bool, "dup path"=w413:path)  [unwired: 8 in, 1 out]
        n380 = And(x=w388, y=w387) -> (x .and. y?=w389:bool)
        n381 = case shown="False" w389 {
          tunnel: w413 -> [_ w441]
          tunnel: [w437 w440] -> w410
          tunnel: [w436 w439] -> w412
          frame False {
            n382 = Read from Text File(prompt (Open existing file)="Info file not found, \nselect by hand") -> (text=w437:string, error out=w436:errorcluster)  [unwired: 3 in, 2 out]
          }
          frame True {
            n383 = Read from Text File(file (use dialog)=w441) -> (text=w440:string, error out=w439:errorcluster)  [unwired: 3 in, 2 out]
          }
        }
        n384 = call "IMAQ Create"("Image Name"="loadedTIFF", "Image Type"=w420) -> ("New Image"=w421:T3)  [unwired: 3 in, 1 out]
        n385 = call "IMAQ ReadFile 2"("File Path"=w396, "error in (no error)"=w425, "Image"=w421) -> ("error out"=w424:errorcluster, "Image Out"=w426:T3)  [unwired: 4 in, 3 out]
        n386 = call <vilib>:"Simple Error Handler.vi"("error in (no error)"=w412) -> ()  [unwired: 4 in, 5 out]
        n387 = Scan From String(format string="Date: %s %s\nx-offset: %.;%f\ny-offset: %.;%f\nImage Width: %f\nResolution: %.;%d\nobj magn: %.;%d\nNA: %.;%f\nDetector Type: %.;%f\nIntegration time [us]: %.;%d\nPower at sample [mW]: %.;%d\nPMT sensitivity: %.;%f\nDAQ readout min: %.;%f\nDAQ readout max: %.;%f\nScanrate (pixels/s): %.;%d\nz-Minimum: %.;%f\nz-stacking: %.;%u\nz-Maximum: %.;%f\nstep-value: %.;%f\nnumber of z steps: %.;%d\nMotor x-pos [µm]: %.;%f\nMotor y-pos [µm]: %.;%f\nMove to z at scan: %.;%u\nXY-Mosaicing: %s\nSlide 1: x-pos: %.;%f; y-pos: %.;%f", input string=w410) -> (output 5=w399:dbl, output 6=w398:i32, output 25=w392:dbl, output 26=w391:dbl)  [unwired: 50 in, 3 out]
        n388 = Divide(x=w399, y=w398) -> (x/y=w405:dbl)
        n389 = global write "xy_stack_global.vi" "FOV Frame (um)"(w399) -> ()
        n390 = local write "FOV Frame"(w399) -> ()
        n391 = global write "xy_stack_global.vi" "Number of pixels Frame"(w398) -> ()
        n392 = local write "No. Pixels Frame"(w398) -> ()
        n393 = call "IMAQ ImageToArray"("error in (no error)"=w424, "Image"=w426) -> ("error out"=w423:errorcluster, "Image Pixels (I16)"=w395:i16[][])  [unwired: 2 in, 3 out]
        n394 = flat-sequence {
          tunnel: w392 -> [w433]
          tunnel: w391 -> [w432]
          tunnel: w401 -> [w431]
          tunnel: w400 -> [w430]
          tunnel: [w430] -> w397
          tunnel: w397 -> [w435]
          frame #0 {
            n395 = local write "X-Minimum"(w433) -> ()
            n396 = local write "Y-Maximum"(w431) -> ()
            n397 = local write "X-Maximum"(w430) -> ()
            n398 = local write "Y-Minimum"(w432) -> ()
          }
          frame #1 {
            n399 = property on="X-Maximum" class="DigNum (strict)"("Val(Sgnl)"=w435) -> ()  [unwired: 2 in, 2 out]
            n400 = local write "loading data"(TRUE ("loading data 2")) -> ()
          }
        }
        n401 = Transpose 2D Array(2D array=w395) -> (transposed array=w394:i16[][])
        n402 = for {
          tunnel: w394 -> [w429] mode=indexing
          tunnel: [w428] -> w393 mode=indexing
          n403 = Reverse 1D Array(array=w429) -> (reversed array=w428:i16[])
        }
        n404 = Array Size(array=w393) -> (size(s)=w404:i32[])
        n405 = Index Array(array=w404, index=0) -> (element=w407:i32)
        n406 = Index Array(array=w404, index=1) -> (element=w406:i32)
        n407 = Multiply(x=w405, y=w406) -> (x*y=w402:dbl)
        n408 = Multiply(x=w405, y=w407) -> (x*y=w403:dbl)
        n409 = Add(x=w392, y=w403) -> (x+y=w400:dbl)
        n410 = Add(x=w391, y=w402) -> (x+y=w401:dbl)
        n411 = local write "Image"(w393) -> ()
      }
      event "compareFOV": Value Change {
        n412 = event-data() -> ()  [unwired: 1 in, 6 out]
        n413 = call "File Dialog5"("pattern (all files)"="*.info") -> ("selected path"=w464:path)  [unwired: 11 in, 3 out]
        n414 = Read from Text File(file (use dialog)=w464) -> (text=w462:string, error out=w465:errorcluster)  [unwired: 3 in, 2 out]
        n415 = call <vilib>:"Simple Error Handler.vi"("error in (no error)"=w465) -> ()  [unwired: 4 in, 5 out]
        n416 = Search and Replace String(input string=w462, search string="Slide ") -> (offset past replacement=w461:i32)  [unwired: 6 in, 3 out]
        n417 = while {
          tunnel: w462 -> [w491]
          shift-right: [w489] -> _
          shift-left: w461 -> [w488]
          shift-right: [w485] -> w458
          shift-left: dbl[] [] ("array") -> [w486]
          shift-right: [w484] -> w450
          shift-left: dbl[] [] -> [w483]
          i -> [w482]
          stop <- w481 stop-if-true
          # "load FOV from info"
          n418 = Scan From String(format string="Slide %u: x-pos: %.;%f; y-pos: %.;%f; z-pos: %.;%f\n", input string=w491, initial scan location=w488) -> (remaining string=w490:string, offset past scan=w489:u32, output 2=w480:dbl, output 3=w479:dbl)  [unwired: 7 in, 1 out]
          n419 = String Length(string=w490) -> (length=w487:i32)
          n420 = Insert Into Array(array=w486, index=w482, new element=w480) -> (w485:dbl[])
          n421 = Insert Into Array(array=w483, new element=w479) -> (w484:dbl[])  [unwired: 1 in]
          n422 = Equal To 0?(x=w487) -> (x = 0?=w481:bool)
        }
        n423 = local read "xLoc ROI"() -> (w457:dbl)
        n424 = local read "yLoc ROI"() -> (w456:dbl)
        n425 = for {
          tunnel: w458 -> [w478] mode=indexing
          tunnel: w457 -> [w476]
          tunnel: w450 -> [w470] mode=indexing
          tunnel: w456 -> [w471]
          tunnel: [w467] -> w454 mode=indexing
          w472 = 64.0 ("y")
          n426 = Add(x=w476, y=w472) -> (x+y=w477:dbl)
          n427 = Subtract(x=w476, y=w472) -> (x-y=w474:dbl)
          n428 = Add(x=w471, y=w472) -> (x+y=w475:dbl)
          n429 = Subtract(x=w471, y=w472) -> (x-y=w473:dbl)
          n430 = In Range and Coerce(upper limit=w477, x=w478, lower limit=w474) -> (In Range?=w469:bool)  [unwired: 1 out]
          n431 = In Range and Coerce(upper limit=w475, x=w470, lower limit=w473) -> (In Range?=w468:bool)  [unwired: 1 out]
          n432 = And(x=w469, y=w468) -> (x .and. y?=w467:bool)
        }
        "Array 2" <- w454
        n433 = Search 1D Array(1D array=w454, element=TRUE) -> (index of element=w449:i32)  [unwired: 1 in]
        n434 = Increment(x=w449) -> (x+1=w448:i32)
        "index 1" <- w448
        n435 = Search 1D Array(1D array=w454, element=TRUE, start index (0)=w448) -> (index of element=w447:i32)
        n436 = Increment(x=w447) -> (x+1=w446:i32)
        "index 2" <- w446
        n437 = Search 1D Array(1D array=w454, element=TRUE, start index (0)=w446) -> (index of element=w445:i32)
        n438 = Increment(x=w445) -> (x+1=w444:i32)
        "index 3" <- w444
        n439 = Search 1D Array(1D array=w454, element=TRUE, start index (0)=w444) -> (index of element=w443:i32)
        n440 = Increment(x=w443) -> (x+1=→"index 4":i32)
      }
      event "SaveROI": Value Change {
        w507 = T2 1 items=["Grayscale (U8)", "Grayscale (I16)", "Grayscale (SGL)", "Complex (CSG)", "RGB (U32)", "HSL (U32)", "RGB (U64)", "Grayscale (U16)"] ("Image Type")
        # "width (px)"
        # "absolute location"
        # "X-loc in PX"
        # "X-location (um, relative)"
        # "px/um"
        # "n_pixels"
        # "load FOV from info"
        n441 = event-data() -> ()  [unwired: 1 in, 6 out]
        n442 = call "File Dialog3"("pattern (all files)"="*.info") -> ("selected path"=w516:path)  [unwired: 11 in, 3 out]
        n443 = Path To String(path=w516) -> (string=w520:string)
        n444 = Read from Text File(file (use dialog)=w516) -> (text=w498:string, error out=w537:errorcluster)  [unwired: 3 in, 2 out]
        n445 = Search and Replace String(input string=w520, search string=".info", replace string="_MOSAIC_FOV_" ("replace string (\"\")")) -> (result string=w502:string, error out=w517:errorcluster)  [unwired: 5 in, 2 out]
        n446 = Search and Replace String(input string=w498, search string="x-offset: ") -> (offset past replacement=w493:i32)  [unwired: 6 in, 3 out]
        n447 = call <vilib>:"Simple Error Handler.vi"("error in (no error)"=w517) -> ()  [unwired: 4 in, 5 out]
        n448 = local read "X-Minimum"() -> (w534:dbl)
        n449 = local read "Y-Minimum"() -> (w533:dbl)
        n450 = Scan From String(format string="x-offset: %.;%f\ny-offset: %.;%f\nImage Width: %f\nResolution: %.;%d\nobj magn: %.;%d\nNA: %.;%f\nDetector Type: %.;%f\nIntegration time [us]: %.;%d\nPower at sample [mW]: %.;%d\nPMT sensitivity: %.;%f\nDAQ readout min: %.;%f\nDAQ readout max: %.;%f\nScanrate (pixels/s): %.;%d\nz-Minimum: %.;%f\nz-stacking: %.;%u\nz-Maximum: %.;%f\nstep-value: %.;%f\nnumber of z steps: %.;%d\nMotor x-pos [µm]: %.;%f\nMotor y-pos [µm]: %.;%f\nMove to z at scan: %.;%u\nXY-Mosaicing: %s", input string=w498, initial scan location=w493) -> (output 3=w496:dbl, output 19=w495:dbl, output 20=w494:dbl)  [unwired: 42 in, 3 out]
        n451 = Format Into String(format string="%u", w496) -> (resulting string=w500:string)  [unwired: 2 in, 1 out]
        n452 = Concatenate Strings(w502, w500, "_um.tiff" ("string")) -> (w503:string)
        n453 = String To Path(string=w503) -> (path=w515:path)
        n454 = Subtract(x=w495, y=w534) -> (x-y=w532:dbl)
        n455 = local read "No. Pixels Frame"() -> (w536:i32)
        n456 = Subtract(x=w494, y=w533) -> (x-y=w531:dbl)
        n457 = call <vilib>:"Simple Error Handler.vi"("error in (no error)"=w537) -> ("error out"=w522:errorcluster)  [unwired: 4 in, 4 out]
        n458 = local read "FOV Frame"() -> (w535:dbl)
        n459 = Divide(x=w536, y=w535) -> (x/y=w530:dbl)
        n460 = Multiply(x=w532, y=w530) -> (x*y=w524:dbl)
        n461 = Multiply(x=w531, y=w530) -> (x*y=w528:dbl)
        n462 = Multiply(x=w496, y=w530) -> (x*y=w525:dbl)
        n463 = call "IMAQ Create"("Image Name"="Image", "Image Type"=w507, "error in (no error)"=w522) -> ("New Image"=w514:T3, "error out"=w512:errorcluster)  [unwired: 2 in]
        n464 = local read "Image"() -> (w529:dbl[][])
        n465 = Subtract(x=w524, y=w525) -> ()  [unwired: 1 out]
        n466 = Array Subset(array=w529, index (row)=w524, length (row)=w525, index (col)=w528, length (col)=w525) -> (w523:dbl[][])
        "Image 2" <- w523
        n467 = for {
          tunnel: w523 -> [w540] mode=indexing
          tunnel: [w539] -> w506 mode=indexing
          n468 = Reverse 1D Array(array=w540) -> (reversed array=w539:dbl[])
        }
        n469 = Transpose 2D Array(2D array=w506) -> (transposed array=w505:dbl[][])
        n470 = call "IMAQ ArrayToImage"("error in (no error)"=w512, "Image Pixels (I16)"=w505, "Image"=w514) -> ("error out"=w511:errorcluster, "Image Out"=w510:T3)  [unwired: 7 in]
        n471 = Array Size(array=w523) -> (size(s)=→"size(s)":i32[])
        n472 = call-poly "IMAQ Write File 2"("error in (no error)"=w511, "TIFF Options"=T1 {"Rows Per Strip"=0, "Photometric"=1, "Compression Type"=3}, "File Path"=w515, "Image"=w510) -> ("error out"=w508:errorcluster, "Image Out (duplicate)"=w509:T3)  [unwired: 6 in]
        n473 = call "IMAQ Dispose"("Image"=w509, "error in (no error)"=w508) -> ("error out"=w521:errorcluster)  [unwired: 4 in]
      }
      event "LoadROIinfo": Value Change {
        # "load FOV from info"
        n474 = event-data() -> ()  [unwired: 1 in, 6 out]
        n475 = call "File Dialog4"("pattern (all files)"="*.info") -> ("selected path"=w546:path)  [unwired: 11 in, 3 out]
        n476 = Read from Text File(file (use dialog)=w546) -> (text=w545:string)  [unwired: 3 in, 3 out]
        n477 = Search and Replace String(input string=w545, search string="x-offset: ") -> (offset past replacement=w541:i32)  [unwired: 6 in, 3 out]
        n478 = Scan From String(format string="x-offset: %.;%f\ny-offset: %.;%f\nImage Width: %f\nResolution: %.;%d\nobj magn: %.;%d\nNA: %.;%f\nDetector Type: %.;%f\nIntegration time [us]: %.;%d\nPower at sample [mW]: %.;%d\nPMT sensitivity: %.;%f\nDAQ readout min: %.;%f\nDAQ readout max: %.;%f\nScanrate (pixels/s): %.;%d\nz-Minimum: %.;%f\nz-stacking: %.;%u\nz-Maximum: %.;%f\nstep-value: %.;%f\nnumber of z steps: %.;%d\nMotor x-pos [µm]: %.;%f\nMotor y-pos [µm]: %.;%f\nMove to z at scan: %.;%u\nXY-Mosaicing: %s", input string=w545, initial scan location=w541) -> (output 19=→"xLoc ROI":dbl, output 20=→"yLoc ROI":dbl)  [unwired: 43 in, 3 out]
      }
      event "Current MAX", "Step Xmax", "Step Ymin", "Step Ymax", "Step Xmin", "Step Size from BS FOV", "Current MIN": Value Change {
        n479 = event-data() -> ()  [unwired: 1 in, 6 out]
        n480 = flat-sequence {
          frame #0 {
            n481 = case shown="True" "Current MAX" {
              frame False {
              }
              frame True {
                n482 = global read "MotorPosition.vi" "Y-Position"() -> (w561:dbl)
                n483 = global read "MotorPosition.vi" "X-Position"() -> (w560:dbl)
                n484 = local write "X-Maximum"(w560) -> ()
                n485 = local write "Y-Maximum"(w561) -> ()
              }
            }
            n486 = case shown="True" "Step Xmin" {
              frame False {
              }
              frame True {
                n487 = local read "X-Minimum"() -> (w563:dbl)
                n488 = local read "Step size X"() -> (w562:dbl)
                n489 = Subtract(x=w563, y=w562) -> (x-y=w564:dbl)
                n490 = local write "X-Minimum"(w564) -> ()
              }
            }
            n491 = case shown="True" "Step Ymin" {
              frame False {
              }
              frame True {
                n492 = local read "Y-Minimum"() -> (w569:dbl)
                n493 = local read "Step size Y"() -> (w568:dbl)
                n494 = Subtract(x=w569, y=w568) -> (x-y=w570:dbl)
                n495 = local write "Y-Minimum"(w570) -> ()
              }
            }
            n496 = case shown="True" "Step Xmax" {
              frame False {
              }
              frame True {
                n497 = local read "X-Maximum"() -> (w572:dbl)
                n498 = local read "Step size X"() -> (w571:dbl)
                n499 = Add(x=w572, y=w571) -> (x+y=w573:dbl)
                n500 = local write "X-Maximum"(w573) -> ()
              }
            }
            n501 = case shown="True" "Step Ymax" {
              frame False {
              }
              frame True {
                n502 = local read "Y-Maximum"() -> (w566:dbl)
                n503 = local read "Step size Y"() -> (w565:dbl)
                n504 = Add(x=w566, y=w565) -> (x+y=w567:dbl)
                n505 = local write "Y-Maximum"(w567) -> ()
              }
            }
            n506 = case shown="True" "Step Size from BS FOV" {
              frame False {
              }
              frame True {
                n507 = global read "xy_stack_global.vi" "FOV Frame (um)"() -> (w559:dbl)
                n508 = local write "Step size X"(w559) -> ()
                n509 = local write "Step size Y"(w559) -> ()
              }
            }
            n510 = case shown="True" "Current MIN" {
              frame False {
              }
              frame True {
                n511 = global read "MotorPosition.vi" "Y-Position"() -> (w558:dbl)
                n512 = global read "MotorPosition.vi" "X-Position"() -> (w557:dbl)
                n513 = local write "Y-Minimum"(w558) -> ()
                n514 = local write "X-Minimum"(w557) -> ()
              }
            }
          }
          frame #1 {
            n515 = local read "X-Maximum"() -> (w574:dbl)
            n516 = property on="X-Maximum" class="DigNum (strict)"("Val(Sgnl)"=w574) -> ()  [unwired: 2 in, 2 out]
          }
        }
      }
    }
  }
  n517 = flat-sequence {
    tunnel: w12 -> [_]
    frame #0 {
      n518 = control-ref of="This VI"() -> (w575:refnum<vi>)
      n519 = invoke class="VI" method="FP.Close"(reference=w575) -> ()  [unwired: 2 in, 3 out]
    }
  }
  n520 = Unregister For Events(event registration refnum=w4, error in=w7) -> (error out=w5:errorcluster)
  n521 = call <vilib>:"Simple Error Handler.vi"("error in (no error)"=w5) -> ()  [unwired: 4 in, 5 out]
